vi "Queue_Driver.vi"(0 "State_and_Data_In":T1, 1 "Max_Queue_Size (-1, unlimited)":i32=-1, 2 "Queue_Name":string, 5 "State_and_Data_In_N":T1[](array[typedef]), 7 "Timeout (-1)":i32, 11 "Error_In":errorcluster, 13 "Queue_Operation_Select":T2=enum."Release_Queue") -> (4 "State_and_Data_Out":T1, 15 "Error_Out":errorcluster)   [LabVIEW 2023]
doc: "Used to send state and event data between the loops"
uses:
  Controls/Queue_Operation_Select.ctl
  Controls/State_and_Data.ctl
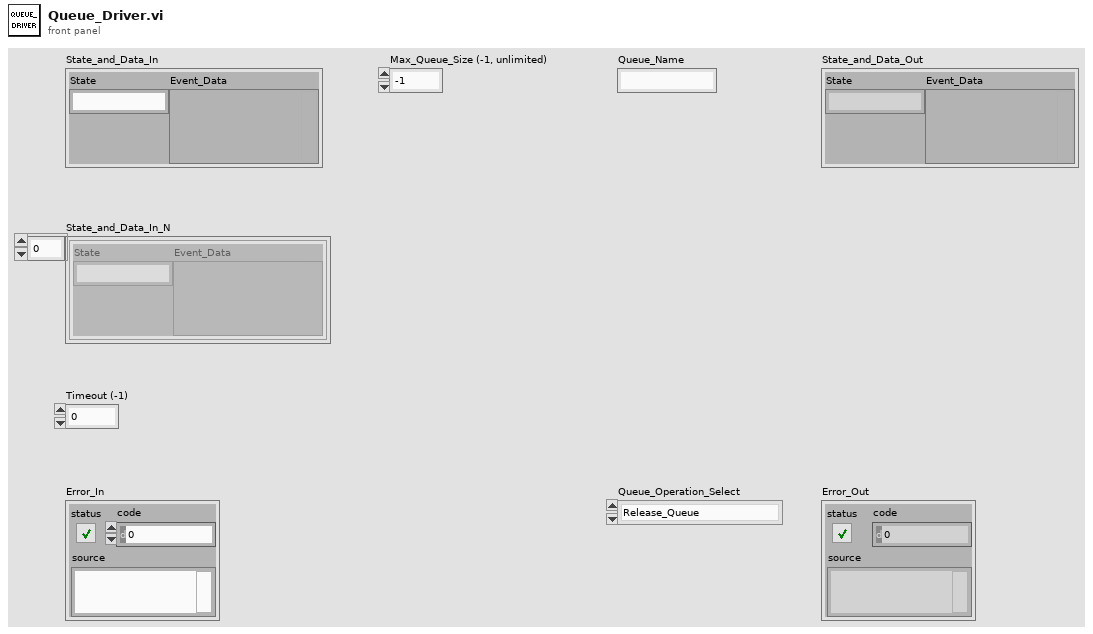
[diagram p1: front panel]
types:
  T1 = typedef "State_and_Data.ctl" = cluster{"State":string, "Event_Data":variant}
  T2 = typedef "Queue_Operation_Select.ctl" = enum16{"Obtain_Queue", "Enqueue", "Enqueue_N", "Enqueue_at_First", "Dequeue", "Flush_Queue", "Release_Queue"}
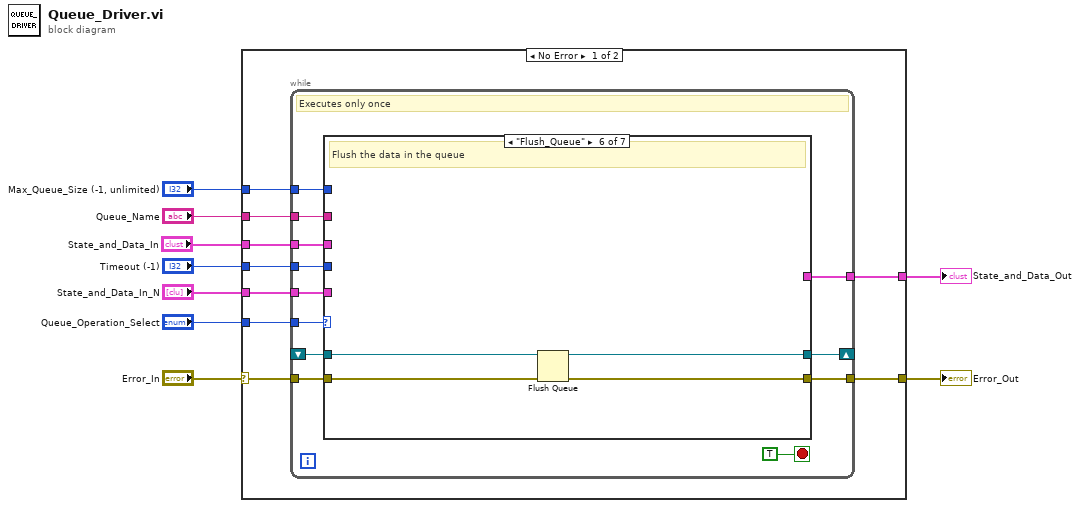
[diagram p0: block diagram]
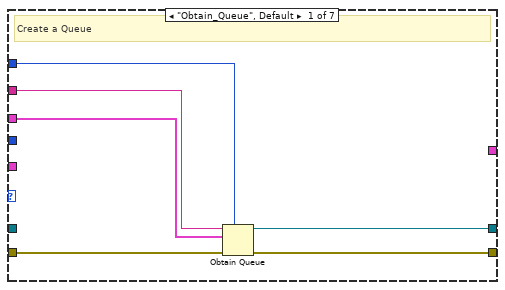
[diagram p2: hidden frame]
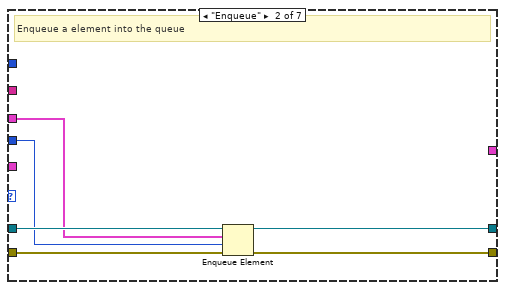
[diagram p3: hidden frame]
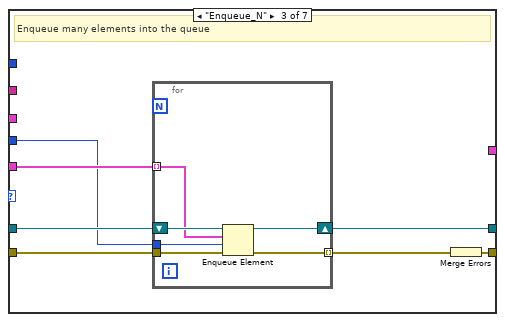
[diagram p4: hidden frame]
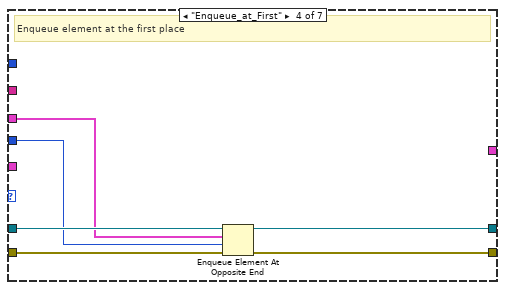
[diagram p5: hidden frame]
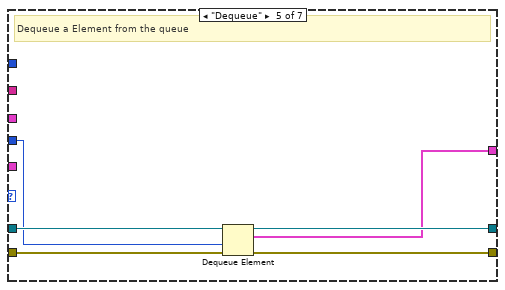
[diagram p6: hidden frame]
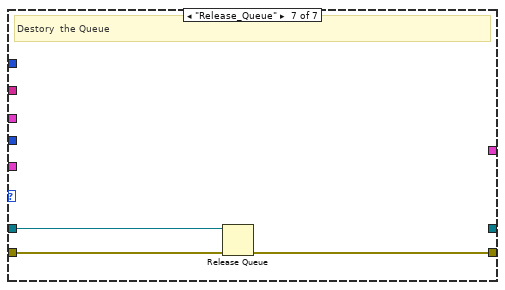
[diagram p7: hidden frame]
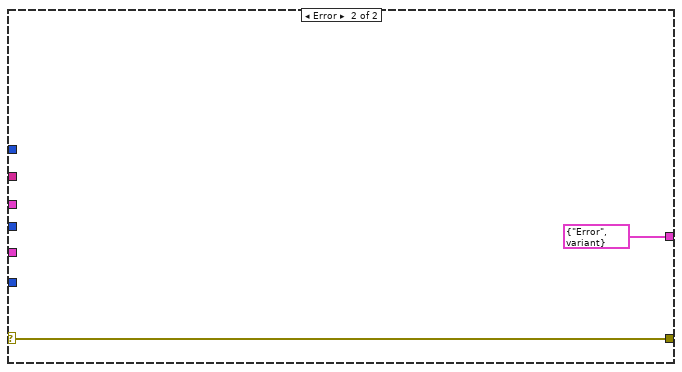
[diagram p8: hidden frame]
diagram:
  n1 = case shown="No Error" "Error_In" {
    selector: "Error_In" -> [w10 w76]
    tunnel: [w18 w76] -> w9
    tunnel: "Queue_Operation_Select" -> [w17 _]
    tunnel: "Queue_Name" -> [w16 _]
    tunnel: "Max_Queue_Size (-1, unlimited)" -> [w15 _]
    tunnel: "Timeout (-1)" -> [w14 _]
    tunnel: "State_and_Data_In" -> [w13 _]
    tunnel: [w12 T1 {"State"="Error", "Event_Data"=variant} ("State_and_Data_In")] -> w3
    tunnel: "State_and_Data_In_N" -> [w11 _]
    frame No Error {
      n2 = while {
        tunnel: w10 -> [w30]
        tunnel: [w29] -> w18
        tunnel: w17 -> [w28]
        tunnel: w16 -> [w27]
        tunnel: w13 -> [w26]
        tunnel: w15 -> [w25]
        shift-right: [w24] -> _
        shift-left: _ -> [w23]
        tunnel: w14 -> [w22]
        tunnel: w11 -> [w21]
        tunnel: [w20] -> w12
        stop <- TRUE stop-if-true
        # "Executes only once"
        n3 = case shown="\"Flush_Queue\"" w28 {
          tunnel: w30 -> [w36 w42 w49 w61 w67 w71 w74]
          tunnel: [w35 w41 w44 w60 w66 w70 w73] -> w29
          tunnel: w27 -> [w34 _ _ _ _ _ _]
          tunnel: w26 -> [w33 w39 _ w58 _ _ _]
          tunnel: w25 -> [w32 _ _ _ _ _ _]
          tunnel: [w31 w37 w45 w56 w63 w68 _] -> w24
          tunnel: w23 -> [_ w40 w46 w59 w65 w69 w72]
          tunnel: w22 -> [_ w38 w43 w57 w64 _ _]
          tunnel: w21 -> [_ _ w47 _ _ _ _]
          tunnel: [_ _ _ _ w62 _ _] -> w20
          frame "Obtain_Queue", Default {
            # "Create a Queue"
            n4 = Obtain Queue(max queue size (-1, unlimited)=w32, name (unnamed)=w34, element data type=w33, error in (no error)=w36) -> (queue out=w31:refnum<queue>, error out=w35:errorcluster)  [unwired: 1 in, 1 out]
          }
          frame "Enqueue" {
            # "Enqueue a element into the queue"
            n5 = Enqueue Element(queue=w40, element=w39, timeout in ms (-1)=w38, error in (no error)=w42) -> (queue out=w37:refnum<queue>, error out=w41:errorcluster)  [unwired: 1 out]
          }
          frame "Enqueue_N" {
            # "Enqueue many elements into the queue"
            n6 = for {
              tunnel: w47 -> [w50] mode=indexing
              tunnel: w49 -> [w55]
              tunnel: [w54] -> w48 mode=indexing
              tunnel: w43 -> [w51]
              shift-right: [w52] -> w45
              shift-left: w46 -> [w53]
              n7 = Enqueue Element(queue=w53, element=w50, timeout in ms (-1)=w51, error in (no error)=w55) -> (queue out=w52:refnum<queue>, error out=w54:errorcluster)  [unwired: 1 out]
            }
            n8 = Merge Errors(w48) -> (w44:errorcluster)
          }
          frame "Enqueue_at_First" {
            # "Enqueue element at the first place"
            n9 = Enqueue Element At Opposite End(queue=w59, element=w58, timeout in ms (-1)=w57, error in (no error)=w61) -> (queue out=w56:refnum<queue>, error out=w60:errorcluster)  [unwired: 1 out]
          }
          frame "Dequeue" {
            # "Dequeue a Element from the queue"
            n10 = Dequeue Element(queue=w65, timeout in ms (-1)=w64, error in (no error)=w67) -> (queue out=w63:refnum<queue>, element=w62:T1, error out=w66:errorcluster)  [unwired: 1 out]
          }
          frame "Flush_Queue" {
            # "Flush the data in the queue"
            n11 = Flush Queue(queue=w69, error in (no error)=w71) -> (queue out=w68:refnum<queue>, error out=w70:errorcluster)  [unwired: 1 out]
          }
          frame "Release_Queue" {
            # "Destory  the Queue"
            n12 = Release Queue(queue=w72, error in (no error)=w74) -> (error out=w73:errorcluster)  [unwired: 1 in, 2 out]
          }
        }
      }
    }
    frame Error {
    }
  }
  "Error_Out" <- w9
  "State_and_Data_Out" <- w3
